vi "Get Result.vi"(6 "Last request":bool, 8 "error in (no error)":errorcluster, 11 "VI Server Recorder in":refnum<class "VI Server Recorder.lvclass">) -> (0 "error out":errorcluster, 2 "Result":refnum<class "Acquired Result.lvclass">, 3 "VI Server Recorder out":refnum<class "VI Server Recorder.lvclass">)   [LabVIEW 2019, in "VI Server Recorder.lvclass"]
uses:
  VI Server Recorder.lvclass
  C:/GitHub/LabActor/Worker/Worker.lvclass
  NHMFL_Core/Libraries/Instruments/Results/Acquired Result/Acquired Result.lvclass
  Worker/Worker.lvclass/Worker.ctl
  <vilib>/express/express signal manip/GetorSetDDTAttributes/Shared VIs/TimeType.ctl
  NHMFL_Core/Libraries/Instruments/Results/Acquired Result/Acquired Result.lvclass/Acquired Result.ctl
  Worker/Read Cycle period.vi
  NHMFL_Core/Libraries/Instruments/Results/Acquired Result/Write Channels.vi
  NHMFL_Core/Libraries/Instruments/Results/Acquired Result/Write Sender.vi
  NHMFL_Core/Libraries/Instruments/Results/Acquired Result/Write Group.vi
  NHMFL_Core/Libraries/Instruments/Results/Acquired Result/Write Final.vi
  <vilib>/express/express signal manip/GetorSetDDTAttributes/Shared VIs/TimeMode Enum to Boolean.vi
  <vilib>/express/express shared/transition.llb/Dynamic To Waveform Array.vi
  <vilib>/express/express signal manip/GetorSetDDTAttributes/Set DDT Attributes/SetT0.vi
  <vilib>/express/express shared/transition.llb/Waveform Array To Dynamic.vi
  Worker/Worker.lvclass
  <vilib>/express/express signal manip/GetorSetDDTAttributes/Set DDT Attributes/Set DDT Properties.xnode
  <vilib>/express/express signal manip/GetorSetDDTAttributes/Shared VIs/GetSetShared.lvlib
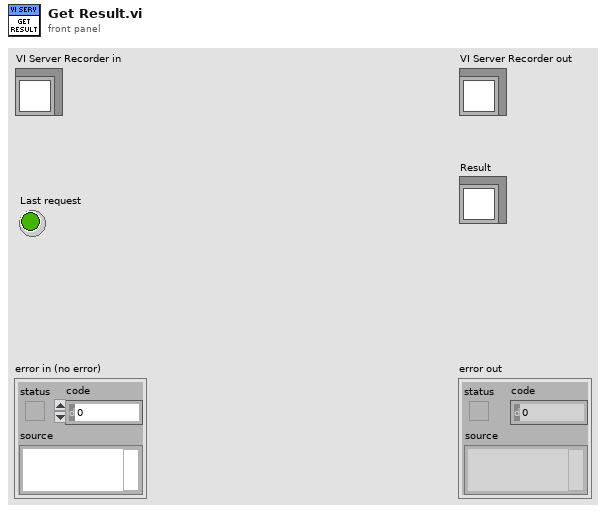
[diagram p1: front panel]
types:
  T1 = typedef "VI Server Configuration.ctl" = cluster{"Machine name (\"\":  open local reference)":string, "Port number (3363)":u16, "Control names":string[], "VI  name":string}
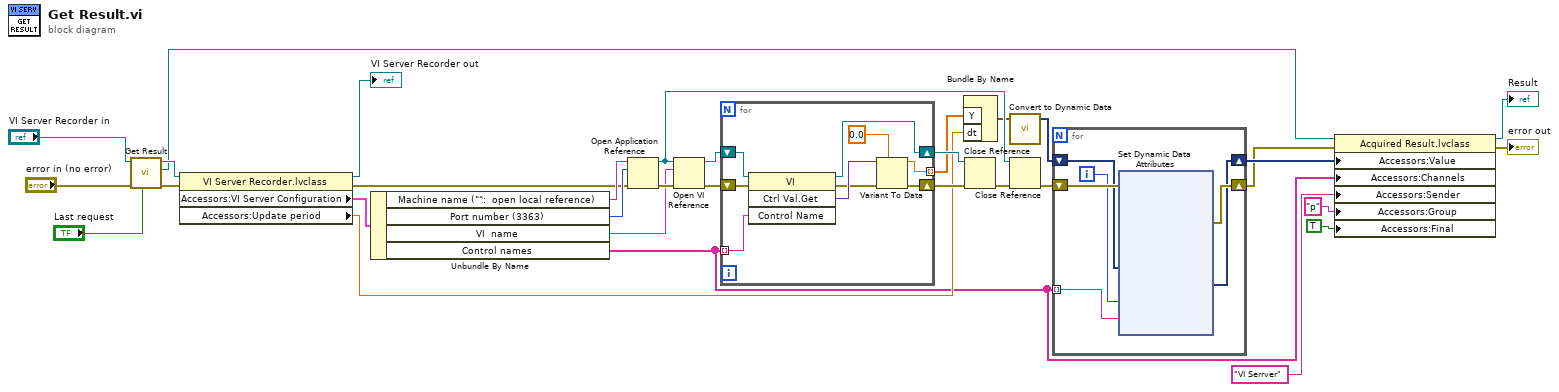
[diagram p0: block diagram]
diagram:
  n1 = call-parent "Get Result.vi"("Last request"="Last request", "error in (no error)"="error in (no error)", "Worker in"="VI Server Recorder in") -> ("error out"=w32:errorcluster, "Result"=w11:refnum<class "Acquired Result.lvclass">, "Worker out"=w26:refnum<class "VI Server Recorder.lvclass">)  [unwired: 6 in]
  n2 = property class="VI Server Recorder.lvclass"(reference=w26, error in=w32) -> (reference out=→"VI Server Recorder out":refnum<class "VI Server Recorder.lvclass">, error out=w20:errorcluster, "Accessors:VI Server Configuration"=w24:T1, "Accessors:Update period"=w13:dbl)
  n3 = Unbundle By Name(w24) -> ("Machine name (\"\":  open local reference)"=w23:string, "Port number (3363)"=w22:u16, "VI  name"=w21:string, "Control names"=w6:string[])
  n4 = Open Application Reference(8:w20, 10:w22, 11:w23) -> (0:w28:errorcluster, 3:w16:refnum<vi>)  [unwired: 1 in]
  n5 = Open VI Reference(application reference (local)=w16, vi path=w21, error in (no error)=w28) -> (vi reference=w27:refnum<vi>, error out=w19:errorcluster)  [unwired: 3 in]
  n6 = for {
    tunnel: w6 -> [w39] mode=indexing
    shift-right: [w35] -> w18
    shift-left: w19 -> [w40]
    shift-right: [w38] -> w17
    shift-left: w27 -> [w41]
    tunnel: [w34] -> w14 mode=indexing
    n7 = invoke class="VI" method="Ctrl Val.Get"(reference=w41, error in=w40, "Control Name"=w39) -> (reference out=w38:refnum<vi>, error out=w36:errorcluster, "Get Control Value Variant"=w37:variant)  [unwired: 1 in, 1 out]
    n8 = Variant To Data(error in=w36, type=0.0, Variant=w37) -> (data=w34:dbl, error out=w35:errorcluster)
  }
  n9 = Bundle By Name("Y"=w14, "dt"=w13) -> (w12:waveform(dbl))  [unwired: 1 in]
  n10 = Close Reference(reference=w17, error in (no error)=w18) -> (error out=w15:errorcluster)
  n11 = call "Convert to Dynamic Data"("Waveform"=w12) -> ("Dynamic Data Type"=w8:dynamicdata)  [unwired: 3 in]
  n12 = Close Reference(reference=w16, error in (no error)=w15) -> (error out=w9:errorcluster)
  n13 = for {
    tunnel: w6 -> [w42] mode=indexing
    shift-right: [w46] -> w1
    shift-left: w9 -> [w47]
    shift-right: [w44] -> w7
    shift-left: w8 -> [w45]
    i -> [w43]
    n14 = xnode "Set Dynamic Data Attributes"("Signals In"=w45, "Signal Index"=w43, "Signal Name"=w42, "error in"=w47) -> ("Signals Out"=w44:dynamicdata, "error out"=w46:errorcluster)  [unwired: 2 in]
  }
  n15 = property class="Acquired Result.lvclass"(reference=w11, error in=w1, "Accessors:Value"=w7, "Accessors:Channels"=w6, "Accessors:Sender"="VI Serrver" ("String"), "Accessors:Group"="p" ("Group"), "Accessors:Final"=TRUE ("Final")) -> (reference out=→"Result":refnum<class "Acquired Result.lvclass">, error out=→"error out":errorcluster)
